vi "XML_FF_readClassList.vi"(8 "error in (no error)":errorcluster, 11 "DOM document in":refnum<k20>) -> (0 "error out":errorcluster, 2 "CLassLabels out":string[](array[string]), 3 "DOM document out":refnum<k20>)   [LabVIEW 2016, in "XML_EEG_Features.lvlib"]
doc: "Прочитать список классов из XML файла"
uses:
  XML_EEG_Features.lvlib
  <vilib>/xml/Close Reference(Node).vi
  <vilib>/xml/NI_XML.lvlib
panel:
  # "This VI is a part of BCI Design library, http://www.ru-bci.org \nCopyright © 2020, Sotnikov Peter, All rights reserved. License: GNU GPLv3"
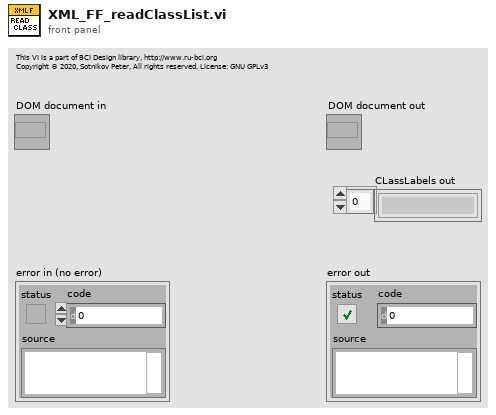
[diagram p1: front panel]
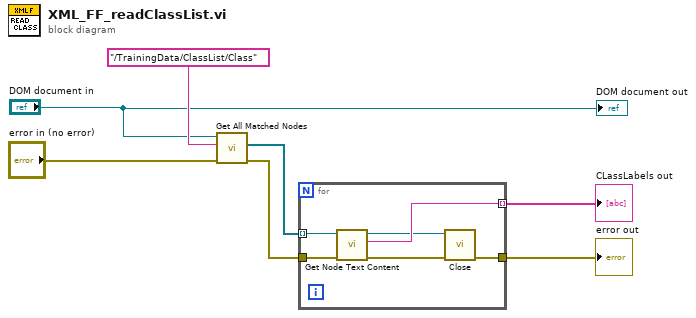
[diagram p0: block diagram]
diagram:
  n1 = call <vilib>:"Get All Matched Nodes.vi"("error in (no error)"="error in (no error)", "XPath expression"="/TrainingData/ClassList/Class", "node in"="DOM document in") -> ("error out"=w5:errorcluster, "node result array"=w6:refnum<k20>[])  [unwired: 6 in, 1 out]
  n2 = for {
    tunnel: w6 -> [w13] mode=indexing
    tunnel: w5 -> [w12]
    tunnel: [w9] -> w2
    tunnel: [w11] -> w3 mode=indexing
    n3 = call <vilib>:"Get Node Text Content.vi"("error in (no error)"=w12, "node in"=w13) -> ("error out"=w10:errorcluster, "node text"=w11:string, "node out"=w8:refnum<k20>)  [unwired: 7 in]
    n4 = call-poly <vilib>:"Close.vi"("error in (no error)"=w10, "node"=w8) -> ("error out"=w9:errorcluster)  [unwired: 7 in]
  }
  "CLassLabels out" <- w3
  "error out" <- w2
  "DOM document out" <- "DOM document in"
